vi "Stopwatch.vi"() -> ()   [LabVIEW 2018]
panel:
  in  "?":bool
  in  "Reset":bool
  out "Seconds":dbl format="%#.3g"
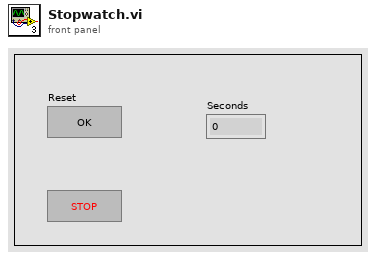
[diagram p1: front panel]
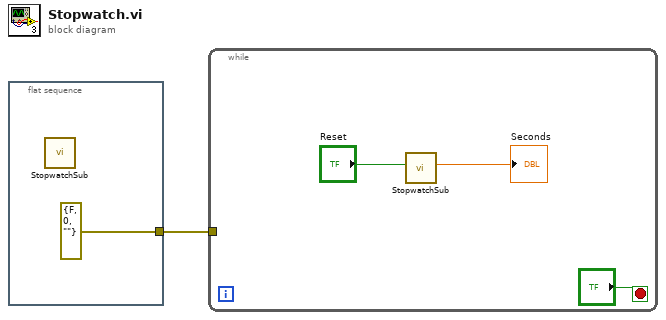
[diagram p0: block diagram]
diagram:
  n1 = flat-sequence {
    tunnel: [errorcluster {"status"=FALSE, "code"=0, "source"=""} ("error constant")] -> w1
    frame #0 {
      n2 = call "StopwatchSub.vi"() -> ()  [unwired: 11 in, 1 out]
    }
  }
  n3 = while {
    tunnel: w1 -> [_]
    stop <- "?" stop-if-true
    n4 = call "StopwatchSub.vi"("Reset"="Reset") -> ("Time(Seconds)"=→"Seconds":dbl)  [unwired: 10 in]
  }
